vi "Basic Dual RT Setup.vi"(8 "error in (no error)":errorcluster, 11 "1553 Unit Test in":refnum<class "Remote Terminal.lvclass">) -> (0 "error out":errorcluster, 3 "1553 Session out":refnum<class "1553 Session.lvclass">)   [LabVIEW 2020, in "Unit Tests.lvlib" / "Remote Terminal.lvclass"]
uses:
  Remote Terminal.lvclass
  1553 Session/1553 Session.lvclass
  Remote Terminal/TypeDefs/RT Configuration.ctl
  Remote Terminal/TypeDefs/RT-RT Timeout.ctl
  Remote Terminal/TypeDefs/Mode Code 17 Sync Configuration.ctl
  Remote Terminal/TypeDefs/RT Timetag Configuration.ctl
  Remote Terminal/TypeDefs/RT Command Config.ctl
  Frames & Messages/TypeDefs/Command Type.ctl
  Frames & Messages/TypeDefs/Command SubAddress.ctl
  Frames & Messages/TypeDefs/Command Word Count.ctl
  Frames & Messages/TypeDefs/Simplified Parameter Data Table.ctl
  Frames & Messages/TypeDefs/Scaling Information.ctl
  Remote Terminal.lvclass/Remote Terminal.ctl
  Remote Terminal/Remote Terminal.lvclass
  C:/Users/MattJ/Desktop/git/bci-1553-labview-api/src/1553 SubComponent/1553 SubComponent.lvclass
  1553 Component/1553 Component.lvclass
  BCI-1553 API.lvlib
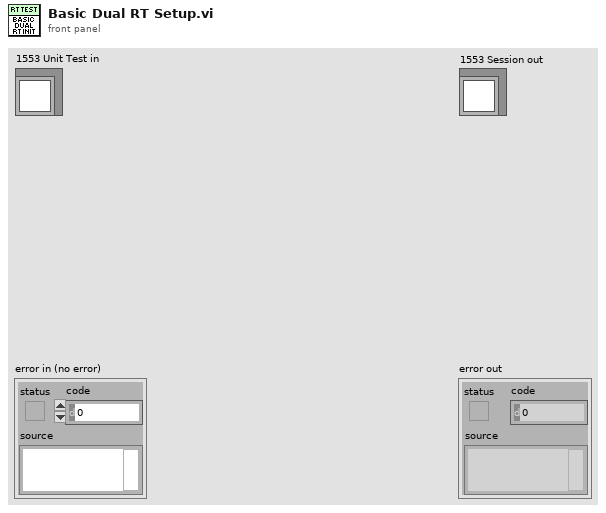
[diagram p1: front panel]
types:
  T1 = typedef "BCI-1553 API.lvlib/Remote Terminal.lvclass/RT Configuration.ctl" = cluster{"RT-RT Timeout":T2, "Inhibit Bus A":bool, "Inhibit Bus B":bool, "Broadcast CMD Invalid":bool, "UnDef MCs Invalid":bool, "Notice 2 Data Storage":bool, "SMCP":bool, "Temp RX Buffer":bool, "Alt BIT Enable":bool, "Auto Bus Shutdown":bool, "MC 16 SR Reset":bool, "MC 17 Sync":T3, "MC 8 Reset":bool, "Remote Terminal Timetag Config":T4}
  T2 = typedef "BCI-1553 API.lvlib/Remote Terminal.lvclass/RT-RT Timeout.ctl" = enum16{"57us", "62us", "100us", "180us"}
  T3 = typedef "BCI-1553 API.lvlib/Remote Terminal.lvclass/Mode Code 17 Sync Configuration.ctl" = enum16{"Sync if Bit 0 = 1", "Sync if Bit 0 = 0", "Sync Unconditionally"}
  T4 = typedef "BCI-1553 API.lvlib/Remote Terminal.lvclass/RT Timetag Configuration.ctl" = enum16{"Disabled", "2us", "4us", "8us", "16us", "32us", "64us"}
  T5 = typedef "BCI-1553 API.lvlib/Remote Terminal.lvclass/RT Command Config.ctl" = cluster{"Command Type":T6, "SubAddress":T7, "Word Count\\Mode Code":T8, "Initial Data":u16[], "Data Fields":T9[]}
  T6 = typedef "BCI-1553 API.lvlib/Command Type.ctl" = enum16{"Transmit", "Receive"}
  T7 = typedef "BCI-1553 API.lvlib/Command SubAddress.ctl" = enum16{"Mode Code", "1", "2", "3", "4", "5", "6", "7", "8", "9", "10", "11", "12", "13", "14", "15", "16", "17", "18", "19", "20", "21", "22", "23", "24", "25", "26", "27", "28", "29", "30"}
  T8 = typedef "BCI-1553 API.lvlib/Command Word Count.ctl" = enum16{"1", "2", "3", "4", "5", "6", "7", "8", "9", "10", "11", "12", "13", "14", "15", "16", "17", "18", "19", "20", "21", "22", "23", "24", "25", "26", "27", "28", "29", "30", "31", "32"}
  T9 = typedef "BCI-1553 API.lvlib/Simplified Parameter Data Table.ctl" = cluster{"Parameter Name":string, "Base Word":u16, "Scaling Info":T10}
  T10 = typedef "BCI-1553 API.lvlib/Scaling Information.ctl" = cluster{"Bit Offset":i32, "Bit Count":i32, "LSB Resolution":dbl, "2's Complement":bool, "Big Endian":bool, "Sign Bit":bool}
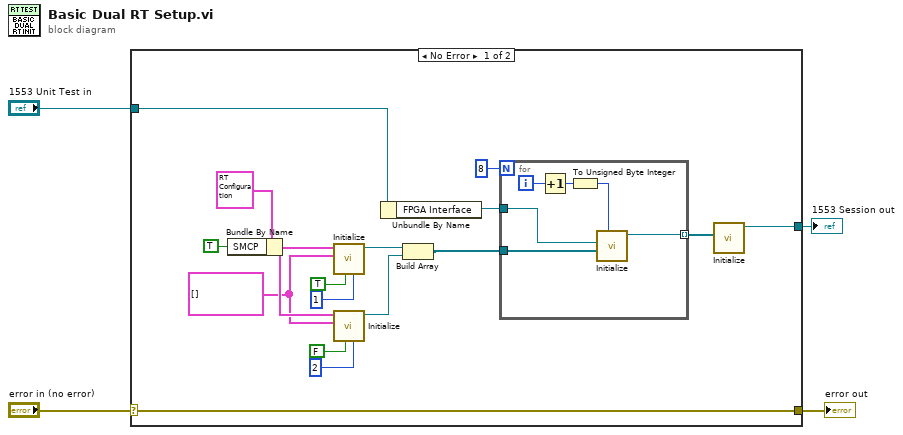
[diagram p0: block diagram]
diagram:
  n1 = case shown="No Error" "error in (no error)" {
    selector: "error in (no error)" -> [w21 w28]
    tunnel: [w21 w28] -> w3
    tunnel: "1553 Unit Test in" -> [w6 _]
    tunnel: [w5 _] -> w1
    frame No Error {
      w8 = T5[] [] ("RT Commands")
      n2 = Bundle By Name(cluster=T1 {"RT-RT Timeout"=enum."57us", "Inhibit Bus A"=FALSE, "Inhibit Bus B"=FALSE, "Broadcast CMD Invalid"=FALSE, "UnDef MCs Invalid"=FALSE, "Notice 2 Data Storage"=FALSE, "SMCP"=FALSE, "Temp RX Buffer"=FALSE, "Alt BIT Enable"=FALSE, "Auto Bus Shutdown"=FALSE, "MC 16 SR Reset"=FALSE, "MC 17 Sync"=enum."Sync if Bit 0 = 1", "MC 8 Reset"=FALSE, "Remote Terminal Timetag Config"=enum."Disabled"} ("RT Configuration"), "SMCP"=TRUE) -> (w19:T1)
      n3 = call "Initialize.vi"("Terminal Address"=u8 1 ("RT Address (0-30)"), "RT 1?"=TRUE, "RT Commands"=w8, "RT Configuration"=w19) -> ("Remote Terminal out"=w13:refnum<class "Remote Terminal.lvclass">)  [unwired: 6 in, 1 out]
      n4 = call "Initialize.vi"("Terminal Address"=u8 2 ("RT Address (0-30)"), "RT 1?"=FALSE, "RT Commands"=w8, "RT Configuration"=w19) -> ("Remote Terminal out"=w12:refnum<class "Remote Terminal.lvclass">)  [unwired: 6 in, 1 out]
      n5 = Unbundle By Name(w6) -> ("FPGA Interface"=w7:refnum<class "FPGA Interface.lvclass">)
      n6 = Build Array(w13, w12) -> (w10:refnum<class "Remote Terminal.lvclass">[])
      n7 = for {
        N: 8 -> [_]
        tunnel: [w25] -> w9 mode=indexing
        tunnel: w10 -> [w24]
        tunnel: w7 -> [w23]
        i -> [w27]
        n8 = Increment(x=w27) -> (x+1=w22:i32)
        n9 = To Unsigned Byte Integer(number=w22) -> (unsigned 8bit integer=w26:u8)
        n10 = call "Initialize.vi"("Component ID (1-8)"=w26, "SubComponents"=w24, "FPGA Interface"=w23) -> ("1553 Component out"=w25:refnum<class "1553 Component.lvclass">)  [unwired: 7 in, 1 out]
      }
      n11 = call "Initialize.vi"("Components"=w9) -> ("1553 Board out"=w5:refnum<class "1553 Session.lvclass">)  [unwired: 9 in, 1 out]
    }
    frame Error {
    }
  }
  "error out" <- w3
  "1553 Session out" <- w1
